vi "Runtime Test.vi"() -> ()   [LabVIEW 2021, in "State Machine tests.lvlib"]
uses:
  State Machine tests.lvlib
  module/execution/State Machine runtime.lvclass
  <vilib>/NI/Tag Bus/dictionary/data dictionary.lvclass/data dictionary.ctl
  <vilib>/NI/Tag Bus/dictionary/lookup polymorphs/locate double.vi
  <vilib>/NI/Tag Bus/table/data polymorphs/read one/read Double.vi
  <vilib>/NI/Tag Bus/table/data polymorphs/write one/write Double.vi
  <vilib>/NI/Tag Bus/dictionary/search/find data index.vi
  <vilib>/NI/Tag Bus/dictionary/search/search string list.vi
  module/configuration/State Machine configuration.lvclass
  C:/Program Files (x86)/National Instruments/LabVIEW 2021/vi.lib/NI/Tag Bus Module Framework/module configuration/TBM module configuration.lvclass
  <vilib>/NI/Tag Bus/dictionary/tag not found.vi
  <vilib>/NI/Tag Bus/dictionary/data dictionary.lvclass
  <vilib>/NI/Tag Bus/table/data table.lvlib
panel:
  in  "output value":dbl=42.0 format="%#_13g"
  out "Input":dbl
  in  "Processing Parameters":dbl
  out "Processing Result":dbl
  out "final error":errorcluster
  out "output error":errorcluster
  out "output lookup error":errorcluster
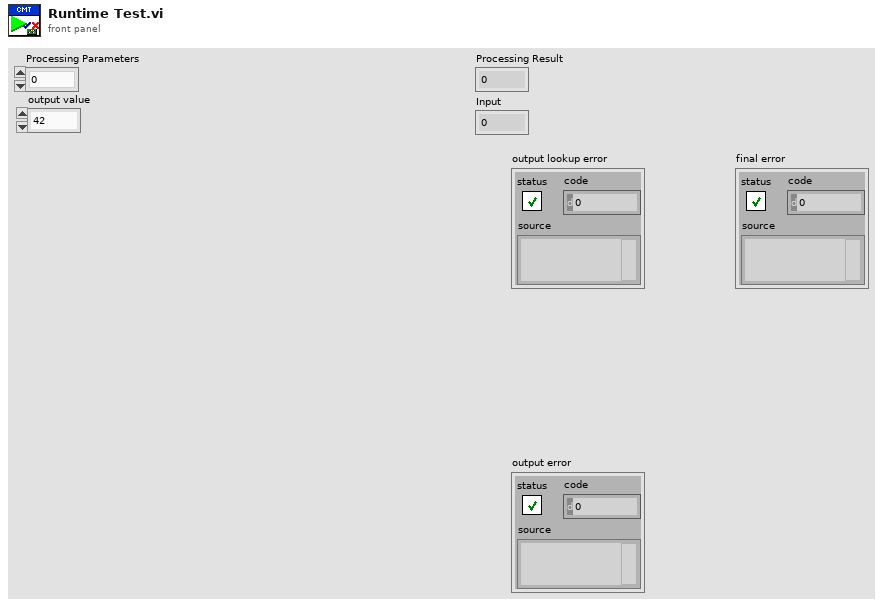
[diagram p1: front panel]
types:
  T1 = typedef "TBM channel.lvclass/data tables.ctl" = cluster{"input data":T2, "processing parameter":T2, "processing result":T2, "output data":T2}
  T2 = typedef "tag bus.lvlib/dictionary table pair.ctl" = cluster{"data dictionary":refnum<class "data dictionary.lvclass">, "data table":T3}
  T3 = typedef "tag bus.lvlib/data table.lvlib/data table.ctl" = cluster{"Double":dbl[], "Single":sgl[], "I64":i64[], "I32":i32[], "I16":i16[], "I8":i8[], "U64":u64[], "U32":u32[], "U16":u16[], "U8":u8[], "Boolean":bool[], "String":string[], "Array of Double":cluster{"DBL Array":dbl[]}[], "Array of Single":cluster{"SGL Array":sgl[]}[], "Array of I64":cluster{"I64 Array":i64[]}[], "Array of I32":cluster{"I32 Array":i32[]}[], "Array of I16":cluster{"I16 Array":i16[]}[], "Array of I8":cluster{"I8 Array":i8[]}[], "Array of U64":cluster{"U64 Array":u64[]}[], "Array of U32":cluster{"U32 Array":u32[]}[], "Array of U16":cluster{"U16 Array":u16[]}[], "Array of U8":cluster{"U8 Array":u8[]}[], "Array of Boolean":cluster{"Boolean Array":bool[]}[], "Array of String":cluster{"String Array":string[]}[]}
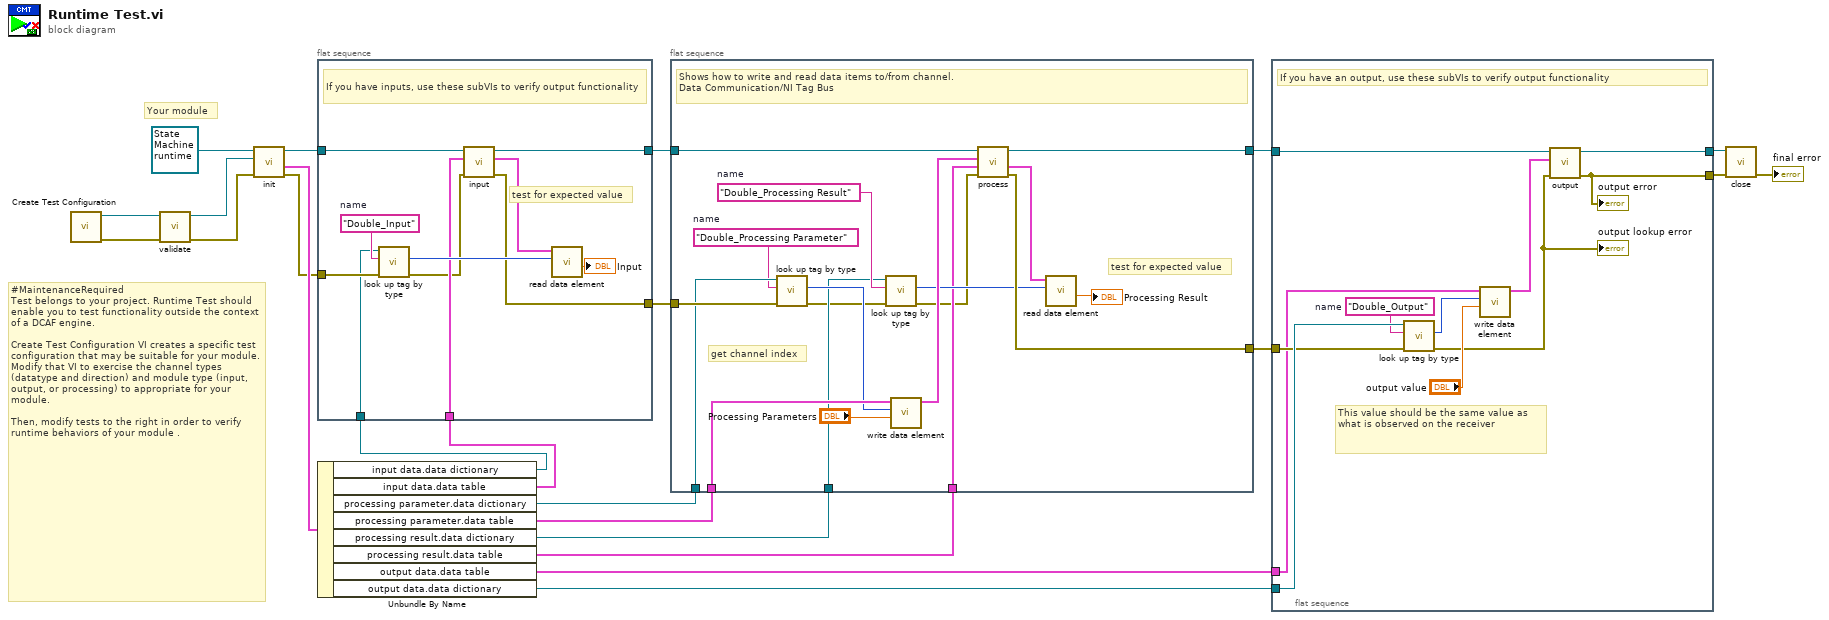
[diagram p0: block diagram]
diagram:
  # "Your module"
  # "#MaintenanceRequired\nTest belongs to your project. Runtime Test should enable you to test functionality outside the context of a DCAF engine. \n\nCreate Test Configuration VI creates a specific test configuration that may be suitable for your module. Modify that VI to exercise the channel types (datatype and direction) and module type (input, output, or processing) to appropriate for your module. \n\nThen, modify tests to the right in order to verify runtime behaviors of your module ."
  n1 = call "Create Test Configuration.vi"() -> ("error out"=w9:errorcluster, "Module"=w11:refnum<class "State Machine configuration.lvclass">)  [unwired: 6 in, 4 out]
  n2 = call-dynamic "validate.vi"("error in"=w9, "fixed channel configuration in"=w11) -> ("error out"=w22:errorcluster, "fixed channel configuration out"=w23:refnum<class "State Machine configuration.lvclass">)  [unwired: 8 in]
  n3 = call-dynamic "init.vi"("error in"=w22, "TBM module configuration in"=w23, "fixed channel runtime in"=refnum<class "State Machine runtime.lvclass"> refnum ("user module")) -> ("error out"=w8:errorcluster, "data allocations"=w21:T1, "fixed channel runtime out"=w6:refnum<class "State Machine runtime.lvclass">)  [unwired: 5 in, 1 out]
  n4 = flat-sequence {
    tunnel: w8 -> [w31]
    tunnel: [w26] -> w7
    tunnel: w6 -> [w34]
    tunnel: [w33] -> w5
    tunnel: w4 -> [w30]
    tunnel: w1 -> [w27]
    frame #0 {
      w32 = "Double_Input"  # name
      # "test for expected value"
      # "If you have inputs, use these subVIs to verify output functionality"
      n5 = call-poly <vilib>:"look up tag by type.vi"("error in"=w31, "name"=w32, "data dictionary in"=w30) -> ("error out"=w25:errorcluster, "index"=w28:i32)  [unwired: 6 in, 1 out]
      n6 = call-dynamic "input.vi"("error in"=w25, "input allocation"=w27, "State Machine runtime in"=w34) -> ("error out"=w26:errorcluster, "input data"=w29:T3, "State Machine runtime out"=w33:refnum<class "State Machine runtime.lvclass">)  [unwired: 6 in]
      n7 = call-poly <vilib>:"read data element.vi"("index"=w28, "data table in"=w29) -> ("value"=→"Input":dbl)  [unwired: 8 in, 1 out]
    }
  }
  n8 = Unbundle By Name(w21) -> ("input data.data dictionary"=w4:refnum<class "data dictionary.lvclass">, "input data.data table"=w1:T3, "processing parameter.data dictionary"=w20:refnum<class "data dictionary.lvclass">, "processing parameter.data table"=w19:T3, "processing result.data dictionary"=w3:refnum<class "data dictionary.lvclass">, "processing result.data table"=w2:T3, "output data.data table"=w12:T3, "output data.data dictionary"=w18:refnum<class "data dictionary.lvclass">)
  n9 = flat-sequence {
    tunnel: w20 -> [w43]
    tunnel: w7 -> [w44]
    tunnel: w19 -> [w52]
    tunnel: [w51] -> w14
    tunnel: [w50] -> w13
    tunnel: w5 -> [w48]
    tunnel: w3 -> [w41]
    tunnel: w2 -> [w39]
    frame #0 {
      w42 = "Double_Processing Parameter"  # name
      w46 = "Double_Processing Result"  # name
      # "test for expected value"
      # "get channel index"
      # "Shows how to write and read data items to/from channel.\nData Communication/NI Tag Bus"
      n10 = call-poly <vilib>:"look up tag by type.vi"("error in"=w44, "name"=w42, "data dictionary in"=w43) -> ("error out"=w38:errorcluster, "index"=w45:i32)  [unwired: 6 in, 1 out]
      n11 = call-poly <vilib>:"look up tag by type.vi"("error in"=w38, "name"=w46, "data dictionary in"=w41) -> ("error out"=w37:errorcluster, "index"=w47:i32)  [unwired: 6 in, 1 out]
      n12 = call-poly <vilib>:"write data element.vi"("value"="Processing Parameters", "index"=w45, "data table in"=w52) -> ("data table out"=w49:T3)  [unwired: 8 in]
      n13 = call-dynamic "process.vi"("error in"=w37, "result allocation"=w39, "parameters"=w49, "State Machine runtime in"=w48) -> ("error out"=w50:errorcluster, "results"=w40:T3, "State Machine runtime out"=w51:refnum<class "State Machine runtime.lvclass">)  [unwired: 4 in, 1 out]
      n14 = call-poly <vilib>:"read data element.vi"("index"=w47, "data table in"=w40) -> ("value"=→"Processing Result":dbl)  [unwired: 8 in, 1 out]
    }
  }
  n15 = flat-sequence {
    tunnel: w18 -> [w63]
    tunnel: [w59] -> w17
    tunnel: [w58] -> w16
    tunnel: w14 -> [w57]
    tunnel: w13 -> [w56]
    tunnel: w12 -> [w55]
    frame #0 {
      w53 = "Double_Output"  # name
      # "This value should be the same value as what is observed on the receiver"
      # "If you have an output, use these subVIs to verify output functionality"
      n16 = call-poly <vilib>:"look up tag by type.vi"("error in"=w56, "name"=w53, "data dictionary in"=w63) -> ("error out"=w54:errorcluster, "index"=w62:i32)  [unwired: 6 in, 1 out]
      "output lookup error" <- w54
      n17 = call-poly <vilib>:"write data element.vi"("value"="output value", "index"=w62, "data table in"=w55) -> ("data table out"=w60:T3)  [unwired: 8 in]
      n18 = call-dynamic "output.vi"("error in"=w54, "output data"=w60, "State Machine runtime in"=w57) -> ("error out"=w58:errorcluster, "State Machine runtime out"=w59:refnum<class "State Machine runtime.lvclass">)  [unwired: 6 in, 1 out]
      "output error" <- w58
    }
  }
  n19 = call-dynamic "close.vi"("error in"=w16, "module in"=w17) -> ("error out"=→"final error":errorcluster)  [unwired: 9 in]
